vi "acquisitionSaveVolume.vi"(1 "folder":string, 2 "volume":u16[][][](array[numeric])) -> ()   [LabVIEW 2017]
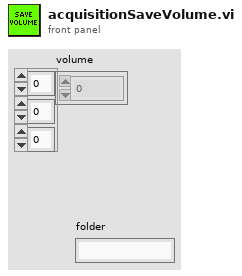
[diagram p1: front panel]
types:
  T1 = enum16{"open", "replace", "create", "open or create", "replace or create", "replace or create with confirmation"}
  T2 = enum16{"big-endian, network order", "native, host order", "little-endian"}
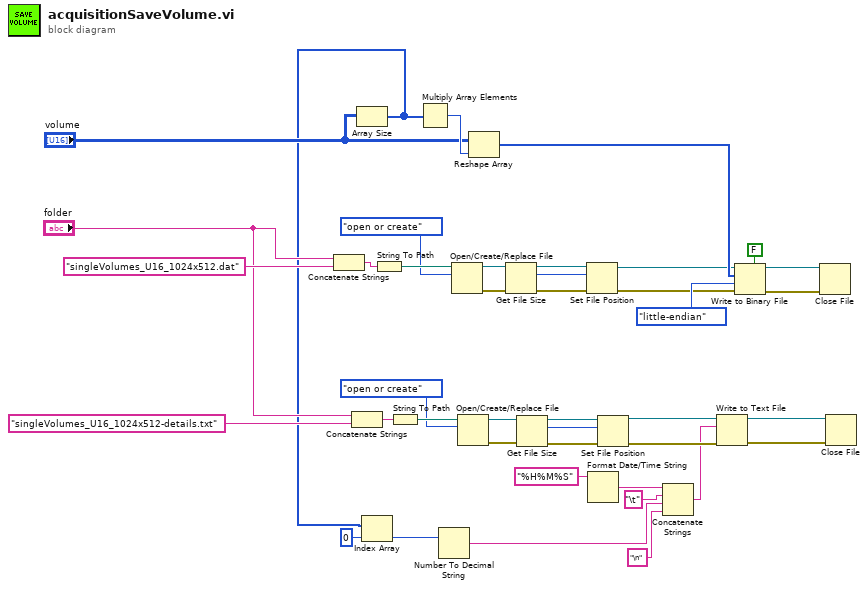
[diagram p0: block diagram]
diagram:
  n1 = Concatenate Strings("folder", "singleVolumes_U16_1024x512.dat" ("string")) -> (w38:string)
  n2 = Concatenate Strings("folder", "singleVolumes_U16_1024x512-details.txt" ("string")) -> (w28:string)
  n3 = Array Size(array="volume") -> (size(s)=w5:i32[])
  n4 = Index Array(array=w5, index=0) -> (element=w3:i32)
  n5 = String To Path(string=w38) -> (path=w37:path)
  n6 = String To Path(string=w28) -> (path=w27:path)
  n7 = Multiply Array Elements(1:w5) -> (0:w41:i32)
  n8 = Number To Decimal String(number=w3) -> (decimal integer string=w2:string)  [unwired: 1 in]
  n9 = Open/Create/Replace File(file path (use dialog)=w37, operation (0:open)=T1."open or create") -> (refnum out=w15:refnum<file>, error out=w14:errorcluster)  [unwired: 4 in, 1 out]
  n10 = Open/Create/Replace File(file path (use dialog)=w27, operation (0:open)=T1."open or create") -> (refnum out=w24:refnum<file>, error out=w25:errorcluster)  [unwired: 4 in, 1 out]
  n11 = Reshape Array("volume", w41) -> (w35:u16[])
  n12 = Get File Size(file=w15, error in=w14) -> (refnum out=w16:refnum<file>, size (in bytes)=w17:i64, 0:w18:errorcluster)
  n13 = Get File Size(file=w24, error in=w25) -> (refnum out=w23:refnum<file>, size (in bytes)=w22:i64, 0:w21:errorcluster)
  n14 = Set File Position(offset (in bytes) (0)=w17, refnum=w16, error in=w18) -> (refnum out=w12:refnum<file>, error out=w13:errorcluster)  [unwired: 1 in]
  n15 = Format Date/Time String(time format string (%c)="%H%M%S") -> (date/time string=w7:string)  [unwired: 2 in]
  n16 = Set File Position(offset (in bytes) (0)=w22, refnum=w23, error in=w21) -> (refnum out=w19:refnum<file>, error out=w20:errorcluster)  [unwired: 1 in]
  n17 = Concatenate Strings(w7, "\t", w2, "\n") -> (w6:string)
  n18 = Write to Text File(file (use dialog)=w19, text=w6, error in=w20) -> (refnum out=w11:refnum<file>, error out=w10:errorcluster)  [unwired: 1 in, 1 out]
  n19 = Write to Binary File(file (use dialog)=w12, data=w35, error in=w13, 5:FALSE ("prepend array or string size? (T)"), 9:T2."little-endian" ("byte order (0:big-endian, network order)")) -> (refnum out=w32:refnum<file>, error out=w31:errorcluster)  [unwired: 1 in, 1 out]
  n20 = Close File(refnum=w32, error in=w31) -> ()  [unwired: 2 out]
  n21 = Close File(refnum=w11, error in=w10) -> ()  [unwired: 2 out]
